vi "ELait03_Query.vi"(7 "String":string, 8 "error in (no error)":errorcluster, 11 "DriverConnect in":T1) -> (0 "error out":errorcluster, 3 "DriverConnect out":T1, 4 "String from device out":string)   [LabVIEW 2018]
uses:
  MOKO_LabViewLibrary/MokoLowLevel/MokoLowLovelControl/MLLC_ConnectCluster.ctl
  MOKO_LabViewLibrary/MokoLowLevel/MokoLowLovelControl/MLLC_InterfaceType.ctl
  MOKO_LabViewLibrary/MokoLowLevel/MokoLowLovelControl/MLLC_OpenedSession.ctl
  MOKO_LabViewLibrary/MokoLowLevel/MokoLowLovelControl/MLLC_InterfaceSettings.ctl
  MOKO_LabViewLibrary/MokoLowLevel/MokoLowLovelControl/MLLC_InterfaceKind.ctl
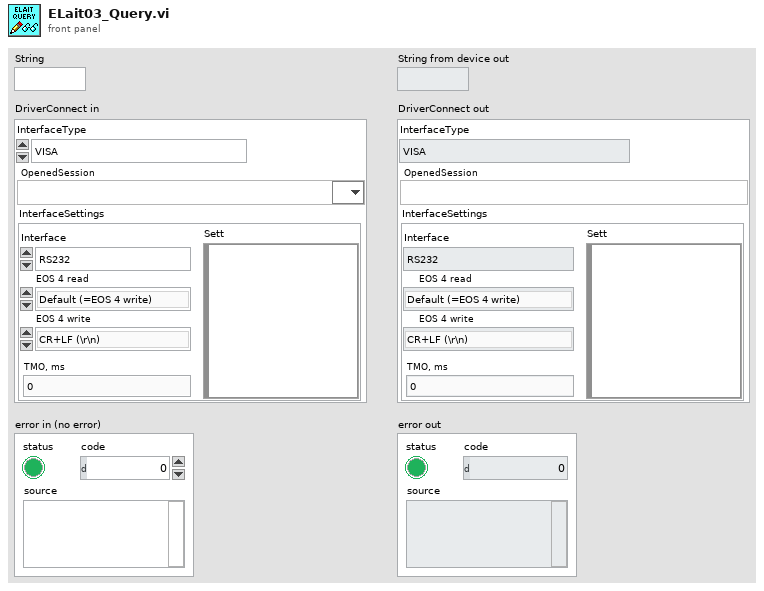
[diagram p1: front panel]
types:
  T1 = typedef "MLLC_ConnectCluster.ctl" = cluster{"InterfaceType":T2, "OpenedSession":T3, "InterfaceSettings":T4}
  T2 = typedef "MLLC_InterfaceType.ctl" = enum16{"VISA", "Prologix USB-GPIB"}
  T3 = typedef "MLLC_OpenedSession.ctl" = refnum<visa-resource-name>
  T4 = typedef "MLLC_InterfaceSettings.ctl" = cluster{"Interface":T5, "EOS 4 read":enum16{"Default (=EOS 4 write)", "CR (\\r)", "LF (\\n)", "None"}, "EOS 4 write":enum16{"CR+LF (\\r\\n)", "CR (\\r)", "LF (\\n)", "None"}, "TMO, ms":i32, "Sett":variant}
  T5 = typedef "MLLC_InterfaceKind.ctl" = enum16{"RS232", "GPIB", "USB", "Ethernet", "another"}
  T6 = typedef "MLLC_Error.ctl" = errorcluster
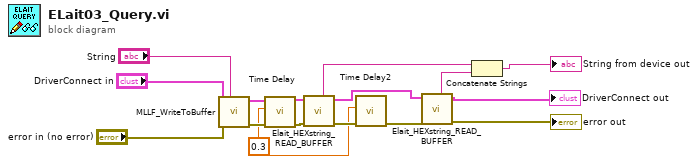
[diagram p0: block diagram]
diagram:
  w8 = 0.3 ("Delay Time (s)")
  n1 = call "MLLF_WriteToBuffer.vi"("String"="String", "error in"="error in (no error)", "DriverConnect in"="DriverConnect in") -> ("error out"=w14:T6, "DriverConnect out"=w12:T1)  [unwired: 5 in]
  n2 = call "Time Delay"("error in (no error)"=w14, "Delay Time (s)"=w8) -> ("error out"=w15:errorcluster)  [unwired: 9 in]
  n3 = call "Elait_HEXstring_READ_BUFFER.vi"("error in"=w15, "DriverConnect in"=w12) -> ("error out"=w9:T6, "DriverConnect out"=w7:T1, "String from device out"=w3:string)  [unwired: 7 in]
  n4 = call "Time Delay2"("error in (no error)"=w9, "Delay Time (s)"=w8) -> ("error out"=w6:errorcluster)  [unwired: 9 in]
  n5 = call "Elait_HEXstring_READ_BUFFER.vi"("error in"=w6, "DriverConnect in"=w7) -> ("error out"=→"error out":T6, "DriverConnect out"=→"DriverConnect out":T1, "String from device out"=w2:string)  [unwired: 7 in]
  n6 = Concatenate Strings(w3, w2) -> (→"String from device out":string)
